vi "Set Badge.vi"(0 "Display State In":T2, 5 "stateIndex":i32, 7 "Badge":T1, 9 "Container State":T6, 11 "error in (no error)":errorcluster, 12 "Visible":bool) -> (4 "Display State Out":T2, 15 "error out":errorcluster)   [LabVIEW 2015, in "FSM Editor.xctl"]
uses:
  FSM Editor.xctl
  <vilib>/_xctls/Container State.ctl
  <vilib>/_xctls/XControlSupport.lvlib
  NodeAdded.ctl
  NodeSelected.ctl
  EdgeEventData.ctl
  Events.ctl
  <vilib>/Utility/miscctls.llb/LVPoint32TypeDef.ctl
  Drag Mode.ctl
  Classes/FSM.Port/FSM.Port.lvclass
  State.vi
  Classes/FSM.Node/Badge.ctl
  Classes/FSM.Node/FSM.Node.lvclass
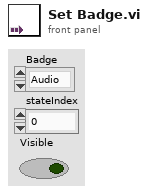
[diagram p1: front panel]
types:
  T1 = typedef "FSM.Node.lvclass/Badge.ctl" = enum16{"Audio", "Visual"}
  T2 = typedef "FSM Editor.xctl/State.vi" = cluster{"snap":bool, "default name":string, "dragStartPoint":T3, "dragMode":T4, "gridsize":dbl, "selectRect":cluster{"left":i16, "top":i16, "right":i16, "bottom":i16}, "events":string[], "cs+/cs-":bool, "insertEdgeAt":string, "insertingEdge":bool, "activePort":refnum<class "FSM.Port.lvclass">, "sourcePort":refnum<class "FSM.Port.lvclass">, "insertionEnd":cluster{"x":i16, "y":i16}, "insertEdgeSpec":string, "nodeIndex":i32, "Events":T5, "action":string}
  T3 = typedef "LVPoint32TypeDef.ctl" = cluster{"Horizontal":i32, "Vertical":i32}
  T4 = typedef "Drag Mode.ctl" = enum16{"Off", "NodePending", "Nodes", "Pan", "Select", "EdgeInsertion", "EdgePoint", "EdgeLabel"}
  T5 = typedef "FSM Editor.xctl/Events.ctl" = cluster{"NodeAdded":refnum<user-event>, "NodeSelected":refnum<user-event>, "EdgeAdded":refnum<user-event>, "EdgeDeleted":refnum<user-event>, "EdgeSelected":refnum<user-event>}
  T6 = typedef "XControlSupport.lvlib/Container State.ctl" = cluster{"Indicator?":bool, "Run Mode?":bool, " Refnum":refnum<vi>}
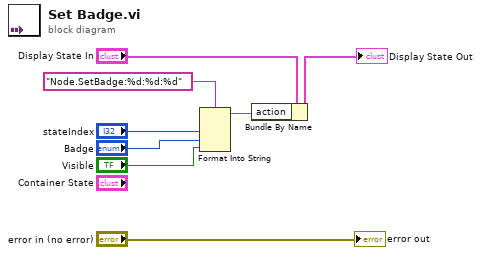
[diagram p0: block diagram]
diagram:
  n1 = Format Into String(format string="Node.SetBadge:%d:%d:%d", "stateIndex", "Badge", "Visible") -> (resulting string=w1:string)  [unwired: 2 in, 1 out]
  n2 = Bundle By Name(cluster="Display State In", "action"=w1) -> (→"Display State Out":T2)
  "error out" <- "error in (no error)"
